vi "node.vi"() -> ()   [LabVIEW 2020]
panel:
  in  "Array":bool[](array[boolean])
  in  "stop":bool
  out "Numeric 5":dbl
  out "Numeric 4":dbl
  out "Numeric 3":dbl
  out "Numeric 2":dbl
  out "Numeric":dbl
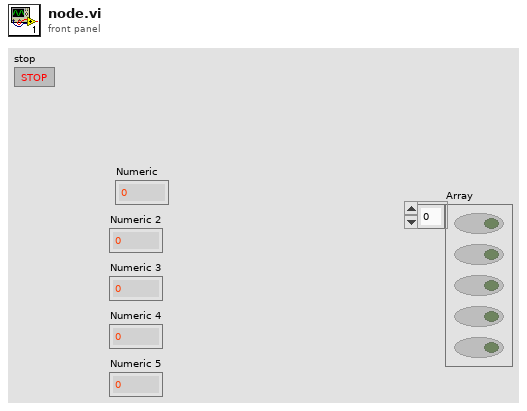
[diagram p1: front panel]
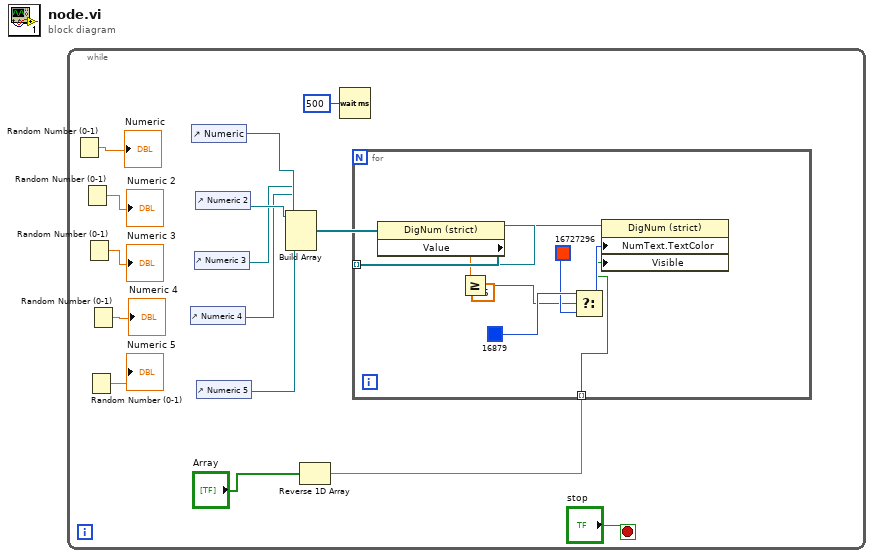
[diagram p0: block diagram]
diagram:
  n1 = while {
    stop <- "stop" stop-if-true
    n2 = Random Number (0-1)() -> (number: 0 to 1=→"Numeric":dbl)
    n3 = Random Number (0-1)() -> (number: 0 to 1=→"Numeric 2":dbl)
    n4 = Random Number (0-1)() -> (number: 0 to 1=→"Numeric 3":dbl)
    n5 = Random Number (0-1)() -> (number: 0 to 1=→"Numeric 5":dbl)
    n6 = Random Number (0-1)() -> (number: 0 to 1=→"Numeric 4":dbl)
    n7 = control-ref of="Numeric 4"() -> (w6:refnum<vi>)
    n8 = control-ref of="Numeric"() -> (w9:refnum<vi>)
    n9 = control-ref of="Numeric 3"() -> (w7:refnum<vi>)
    n10 = control-ref of="Numeric 2"() -> (w8:refnum<vi>)
    n11 = control-ref of="Numeric 5"() -> (w5:refnum<vi>)
    n12 = Build Array(w9, w8, w7, w6, w5) -> (w4:refnum<vi>[])
    n13 = Reverse 1D Array(array="Array") -> (reversed array=w1:bool[])
    n14 = Wait (ms)(milliseconds to wait=u32 500) -> ()  [unwired: 1 out]
    n15 = for {
      tunnel: w4 -> [w24] mode=indexing
      tunnel: w1 -> [w16] mode=indexing
      n16 = property class="DigNum (strict)"(reference=w24) -> (reference out=w21:refnum<vi>, "Value"=w22:dbl)  [unwired: 1 in, 1 out]
      n17 = Greater Or Equal?(x=w22, y=0.5) -> (x >= y?=w18:bool)
      n18 = Select(t=u32 16879 ("Numeric Text.Text Colors:Text Color"), s=w18, f=u32 16727296 ("Numeric Text.Text Colors:Text Color")) -> (s? t:f=w17:u32)
      n19 = property class="DigNum (strict)"(reference=w21, "NumText.TextColor"=w17, "Visible"=w16) -> ()  [unwired: 1 in, 2 out]
    }
  }
